vi "ScanAction.vi"(8 "error in (no error)":errorcluster caption="entrée d'erreur (pas d'erreur)", 9 "IndicePoint":i32, 10 "Dir":bool, 11 "DK240 In":refnum<class "DK240.lvclass"> caption="DNL_LabVIEW Object in") -> (0 "error out":errorcluster caption="sortie d'erreur", 2 "ScanParsOut":dbl[](array[numeric]), 3 "DK240 Out":refnum<class "DK240.lvclass"> caption="DNL_LabVIEW Object out")   [LabVIEW 2019, in "DK240.lvclass"]
uses:
  DK240.lvclass
  C:/Programmes Labview/LabScanV1A/DevicesClass/BaseDevice/BaseDevice.lvclass
  DK240.lvclass/DK240.ctl
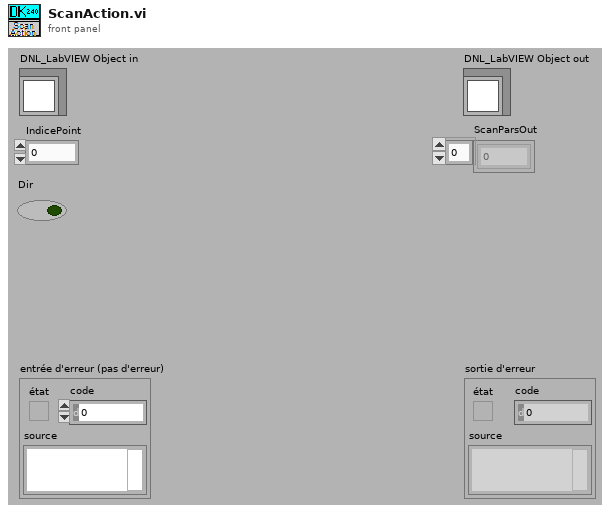
[diagram p1: front panel]
types:
  T1 = typedef "DK240.lvclass/DK240_Func.ctl" = enum16{"Wavelenght (nm)"}
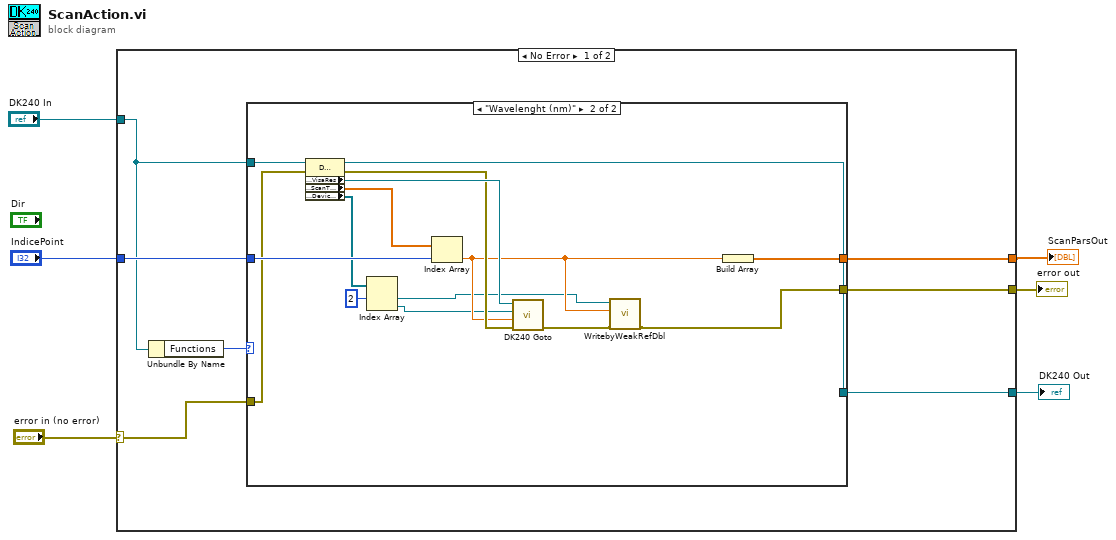
[diagram p0: block diagram]
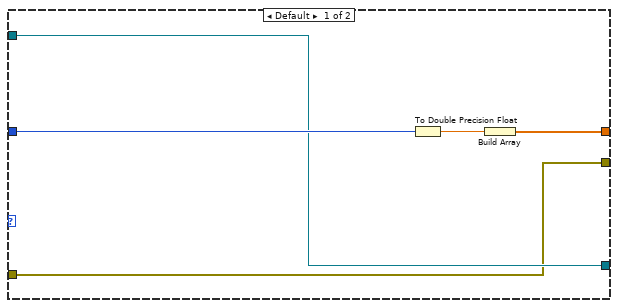
[diagram p2: hidden frame]
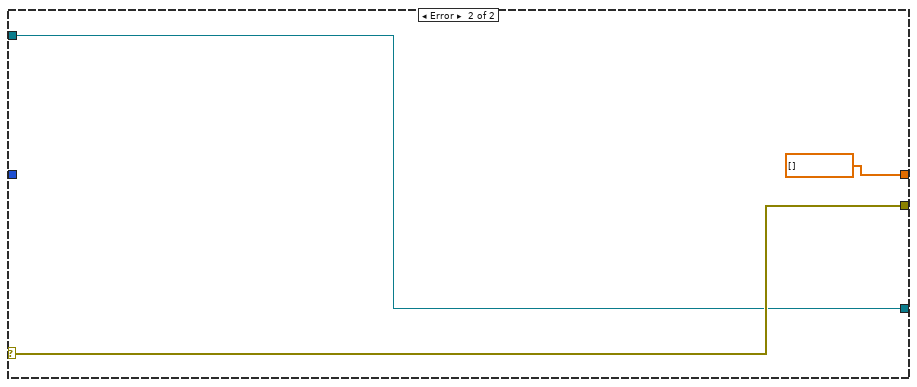
[diagram p3: hidden frame]
diagram:
  n1 = case shown="No Error" "error in (no error)" {
    selector: "error in (no error)" -> [w10 w36]
    tunnel: "DK240 In" -> [w11 w35]
    tunnel: [w9 dbl[] []] -> w1
    tunnel: [w8 w36] -> w4
    tunnel: [w7 w35] -> w3
    tunnel: "IndicePoint" -> [w12 _]
    frame No Error {
      n2 = Unbundle By Name(w11) -> ("Functions"=w13:T1)
      n3 = case shown="\"Wavelenght (nm)\"" w13 {
        tunnel: [w14 w31] -> w9
        tunnel: w12 -> [w18 w33]
        tunnel: [w16 w30] -> w7
        tunnel: w11 -> [w16 w32]
        tunnel: w10 -> [w15 w29]
        tunnel: [w15 w24] -> w8
        frame Default {
          n4 = To Double Precision Float(number=w18) -> (double precision float=w17:dbl)
          n5 = Build Array(w17) -> (w14:dbl[])
        }
        frame "Wavelenght (nm)" {
          n6 = property class="DK240.lvclass"(reference=w32, error in=w29) -> (reference out=w30:refnum<class "DK240.lvclass">, error out=w26:errorcluster, "Accessor:VisaRes"=w27:refnum<visa-resource-name>, "Accessor:ScanTable"=w28:dbl[], "Accessor:DeviceCtrl"=w22:refnum<vi>[])
          n7 = Index Array(array=w22, index #1=2 ("indice")) -> (element #1=w19:refnum<vi>, element #2=w20:refnum<vi>)  [unwired: 1 in]
          n8 = Index Array(array=w28, index=w33) -> (element=w23:dbl)
          n9 = call <userlib>:"DK240 Goto.vi"("error in"=w26, "Wavelenght"=w23, "MovingRef"=w20, "Port"=w27) -> ("error out"=w25:errorcluster)  [unwired: 2 in, 2 out]
          n10 = call <userlib>:"WritebyWeakRefDbl.vi"("error in"=w25, "Valeur"=w23, "Control Ref"=w19) -> ("error out"=w24:errorcluster)  [unwired: 8 in]
          n11 = Build Array(w23) -> (w31:dbl[])
        }
      }
    }
    frame Error {
    }
  }
  "error out" <- w4
  "DK240 Out" <- w3
  "ScanParsOut" <- w1
